vi "update.name.request.vi"(8 "error in":errorcluster, 10 "Name":string, 11 "event":refnum<class "event.lvclass">) -> (0 "error out":errorcluster, 3 "request":string)   [LabVIEW 2020, in "event.lvclass"]
uses:
  event.lvclass
  event.lvclass/event.ctl
  <vilib>/JDP Science/JSONtext/LVClass Serializer/JSONtext LVClass Serializer.lvclass
  d06e21f4-b86b-41cf-b884-0b757daf40c2.vi
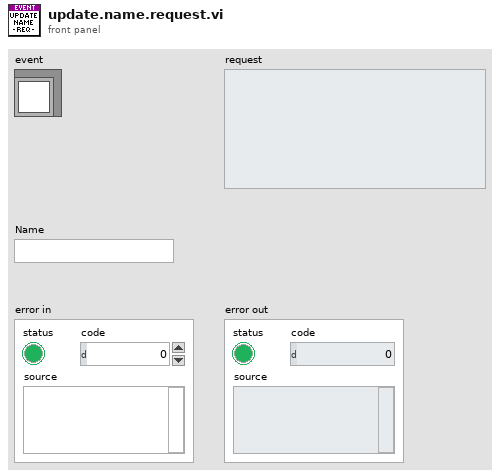
[diagram p1: front panel]
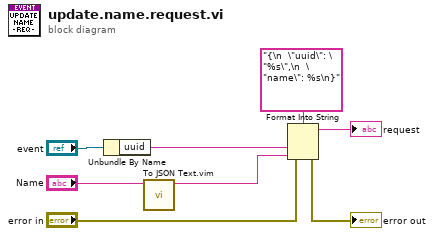
[diagram p0: block diagram]
diagram:
  n1 = Unbundle By Name("event") -> ("uuid"=w6:string)
  n2 = call "To JSON Text.vim"("Anything"="Name") -> ("<JSON>"=w1:string)  [unwired: 9 in, 1 out]
  n3 = Format Into String(format string="{\n  \"uuid\": \"%s\",\n  \"name\": %s\n}", error in="error in", w6, w1) -> (resulting string=→"request":string, error out=→"error out":errorcluster)  [unwired: 1 in]
